vi "init.vi"(0 "Camera in":refnum<class "Camera.lvclass">, 1 "interface":u16(ring)=65535 items=["FireWire"=1, "GenICam"=3, "GigE"=5, "USB"=6, "CameraLinkME4"=7, "USB3"=8, "CLHS"=11, "All"=65535], 2 "serial":u32=4294967295 format="%0d", 3 "error in (no error)":errorcluster) -> (7 "Camera out":refnum<class "Camera.lvclass">, 10 "error out":errorcluster)   [LabVIEW 2019, in "Camera.lvclass"]
doc: "Opens communication and initializes a camera. With the \"All interfaces\" option, this VI will scan through all possible interfaces until it finds a connected camera. Alternatively, the interface can be specified. An error is generated if no camera is found. The camera is set to a defult configuration by this VI."
uses:
  Camera.lvclass
  Camera.lvclass/Camera.ctl
  pco.sdk/Structures/Structures.lvlib
  pco.sdk/CameraAccess/CameraAccess.lvlib
  pco.sdk/CameraDescription/CameraDescription.lvlib
  pco.sdk/GeneralCameraStatus/GeneralCameraStatus.lvlib
  pco.convert/Convert.lvlib
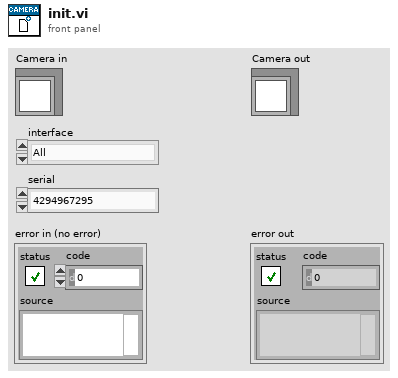
[diagram p1: front panel]
types:
  T1 = cluster{"wCamType":u16, "wCamSubType":u16, "dwSerialNumber":u32, "dwHWVersion":u32, "dwFWVersion":u32, "InterfaceType":u16, "PCO_FW_Vers":cluster{"wDeviceNum":u16, "PCO_SC2_Firmware_DESC":cluster{"szName":string, "bMinorRev":u8, "bMajorRev":u8, "wVariant":u16}[]}, "PCO_HW_Vers":cluster{"wBoardNum":u16, "PCO_SC2_Hardware_DESC":cluster{"szName":string, "wBatchNo":u16, "wRevision":u16, "wVariant":u16}[]}}
  T2 = cluster{"wSensorTypeDESC":u16, "wSensorSubTypeDESC":u16, "wMaxHorzResStdDESC":u16, "wMaxVertResStdDESC":u16, "wMaxHorzResExtDESC":u16, "wMaxVertResExtDESC":u16, "wDynResDESC":u16, "wMaxBinHorzDESC":u16, "wBinHorzSteppingDESC":u16, "wMaxBinVertDESC":u16, "wBinVertSteppingDESC":u16, "wRoiHorStepsDESC":u16, "wRoiVertStepsDESC":u16, "wNumADCsDESC":u16, "wMinSizeHorzDESC":u16, "dwPixelRateDESC":u32[], "wConvFactDESC":u16[], "sCoolingSetpoints":i16[], "wSoftRoiHorStepsDESC":u16, "wSoftRoiVertStepsDESC":u16, "wIRDESC":u16, "wMinSizeVertDESC":u16, "dwMinDelayDESC":u32, "dwMaxDelayDESC":u32, "dwMinDelayStepDESC":u32, "dwMinExposureDESC":u32, "dwMaxExposureDESC":u32, "dwMinExposureStepDESC":u32, "dwMinDelayIRDESC":u32, "dwMaxDelayIRDESC":u32, "dwMinExposureIRDESC":u32, "dwMaxExposureIRDESC":u32, "wTimeTableDESC":u16, "wDoubleImageDESC":u16, "sMinCoolSetDESC":i16, "sMaxCoolSetDESC":i16, "sDefaultCoolSetDESC":i16, "wPowerDownModeDESC":u16, "wOffsetRegulationDESC":u16, "wColorPatternDESC":u16, "wPatternTypeDESC":u16, "wNumCoolingSetpoints":u16, "dwGeneralCapsDESC1":u32, "dwGeneralCapsDESC2":u32, "dwExtSyncFrequency":u32[], "dwGeneralCapsDESC3":u32, "dwGeneralCapsDESC4":u32}
  T3 = cluster{"sharpen":bool, "adaptive_sharpen":bool, "flip_vertical":bool, "auto_minmax":bool, "add_conv_flags":u32, "min_limit":u16, "max_limit":u16, "gamma":dbl, "contrast":i32, "pco_debayer_algorithm":bool, "color_temperature":i32, "color_saturation":i32, "color_vibrance":i32, "color_tint":i32, "lut_file":path}
  T4 = cluster{"wInterfaceType":u16, "wCameraNumber":u16, "wCameraNumAtInterface":u16, "wOpenFlags":u16[], "dwOpenFlags":u32[], "wOpenPtr":u64[]}
  T5 = cluster{"iConversionFactor":i32, "iDataBits":i32, "iSensorInfoBits":i32, "iDarkOffset":i32, "strColorCoeff":dbl[], "iCamNum":i32, "hCamera":u64}
  T6 = enum16{"Undefined", "Mono8", "Mono16", "BGRA8", "RGBA8", "BGRA16", "RGBA16", "CompressedMono8"}
  T7 = map{enum16{"Undefined", "Mono8", "Mono16", "BGRA8", "RGBA8", "BGRA16", "RGBA16", "CompressedMono8"}, bool}
  T8 = map{enum16{"Undefined", "Mono8", "Mono16", "BGRA8", "RGBA8", "BGRA16", "RGBA16", "CompressedMono8"}, cluster{"sharpen":bool, "adaptive_sharpen":bool, "flip_vertical":bool, "auto_minmax":bool, "add_conv_flags":u32, "min_limit":u16, "max_limit":u16, "gamma":dbl, "contrast":i32, "pco_debayer_algorithm":bool, "color_temperature":i32, "color_saturation":i32, "color_vibrance":i32, "color_tint":i32, "lut_file":path}}
  T9 = map{enum16{"Undefined", "Mono8", "Mono16", "BGRA8", "RGBA8", "BGRA16", "RGBA16", "CompressedMono8"}, u64}
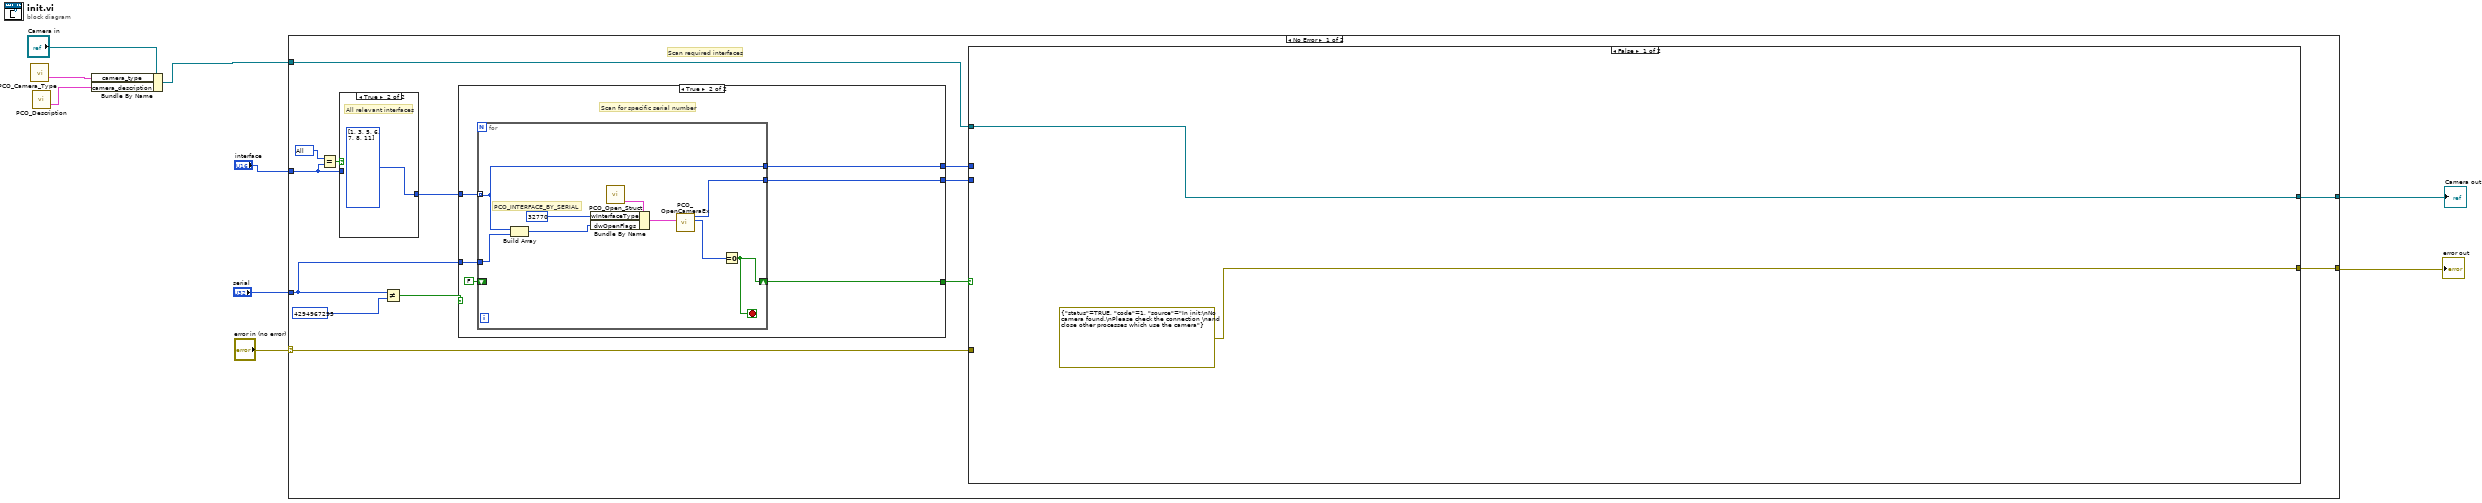
[diagram p0: block diagram]
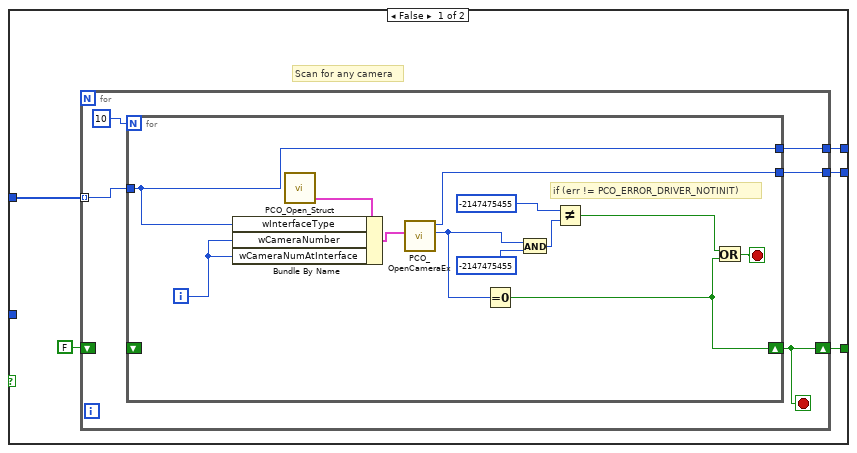
[diagram p2: hidden frame]
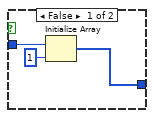
[diagram p3: hidden frame]
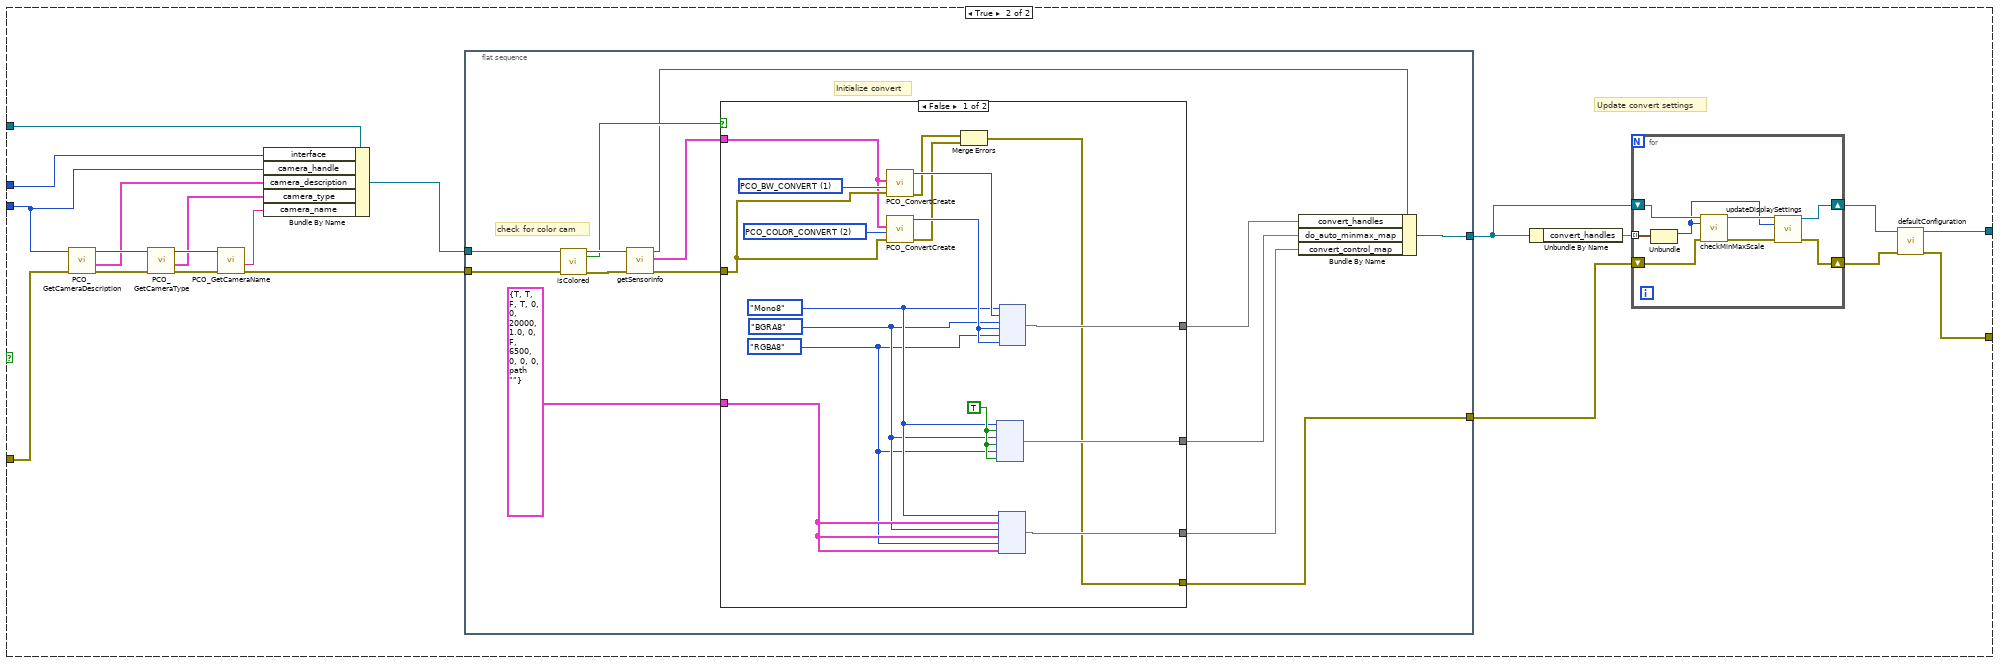
[diagram p4: hidden frame]
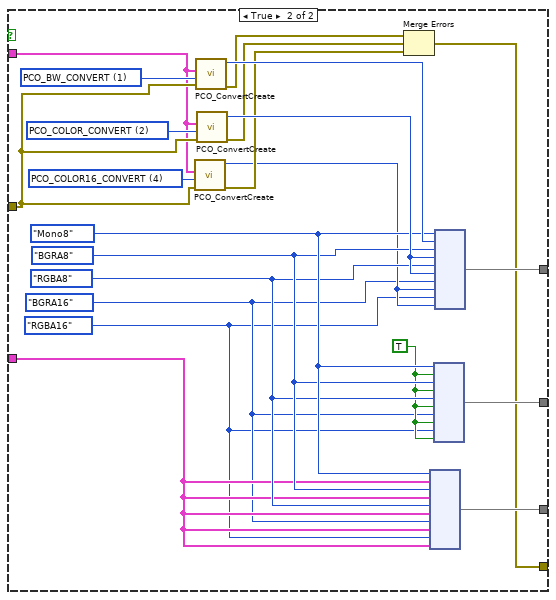
[diagram p5: hidden frame]
diagram:
  n1 = call "PCO_Camera_Type.vi"() -> ("PCO_CameraType"=w5:T1)  [unwired: 4 in, 3 out]
  n2 = call "PCO_Description.vi"() -> ("PCO_Description"=w4:T2)  [unwired: 4 in, 3 out]
  n3 = Bundle By Name(cluster="Camera in", "camera_type"=w5, "camera_description"=w4) -> (w2:refnum<class "Camera.lvclass">)
  n4 = case shown="No Error" "error in (no error)" {
    selector: "error in (no error)" -> [w15 w149]
    tunnel: [w21 w149] -> w8
    tunnel: [w19 w148] -> w7
    tunnel: w2 -> [w20 w148]
    tunnel: "interface" -> [w17 _]
    tunnel: "serial" -> [w10 _]
    frame No Error {
      w13 = u16 65535 items=["FireWire"=1, "GenICam"=3, "GigE"=5, "USB"=6, "CameraLinkME4"=7, "USB3"=8, "CLHS"=11, "All"=65535] ("interface")
      # "Scan required interfaces"
      n5 = Equal?(x=w13, y=w17) -> (x = y?=w18:bool)
      n6 = case shown="True" w18 {
        tunnel: w17 -> [w63 _]
        tunnel: [w61 u16[] [1, 3, 5, 6, 7, 8, 11]] -> w16
        frame False {
          n7 = Initialize Array(w63, 1 ("dimension size")) -> (w61:u16[])
        }
        frame True {
          # "All relevant interfaces"
        }
      }
      n8 = Not Equal?(x=w10, y=u32 4294967295) -> (x != y?=w11:bool)
      n9 = case shown="True" w11 {
        tunnel: [w28 w46] -> w23
        tunnel: [w27 w48] -> w22
        tunnel: w16 -> [w25 w50]
        tunnel: [w24 w47] -> w14
        tunnel: w10 -> [_ w49]
        frame False {
          # "Scan for any camera"
          n10 = for {
            shift-right: [w31] -> w28
            shift-left: FALSE -> [_]
            tunnel: w25 -> [w30] mode=indexing
            tunnel: [w32] -> w27
            tunnel: [w29] -> w24
            stop <- w31 stop-if-true
            n11 = for {
              N: 10 -> [_]
              tunnel: w30 -> [w34]
              shift-right: [w41] -> w31
              shift-left: _ -> [_]
              tunnel: [w39] -> w32
              tunnel: [w34] -> w29
              i -> [w35]
              stop <- w40 stop-if-true
              # "if (err != PCO_ERROR_DRIVER_NOTINIT)"
              n12 = call "PCO_Open_Struct.vi"() -> ("PCO_Open_Struct"=w45:T4)  [unwired: 4 in, 4 out]
              n13 = Bundle By Name(cluster=w45, "wInterfaceType"=w34, "wCameraNumber"=w35, "wCameraNumAtInterface"=w35) -> (w44:T4)
              n14 = call "PCO_OpenCameraEx.vi"("strOpenStruct"=w44) -> ("ErrorMessage"=w36:i32, "ph out"=w39:u64)  [unwired: 8 in, 1 out]
              n15 = Equal To 0?(x=w36) -> (x = 0?=w41:bool)
              n16 = And(x=w36, y=-2147475455 ("x")) -> (x .and. y?=w38:i32)
              n17 = Not Equal?(x=-2147475455, y=w38) -> (x != y?=w42:bool)
              n18 = Or(x=w42, y=w41) -> (x .or. y?=w40:bool)
            }
          }
        }
        frame True {
          # "Scan for specific serial number"
          n19 = for {
            shift-right: [w52] -> w46
            shift-left: FALSE -> [_]
            tunnel: w50 -> [w53] mode=indexing
            tunnel: w49 -> [w56]
            tunnel: [w54] -> w48
            tunnel: [w53] -> w47
            stop <- w52 stop-if-true
            # "PCO_INTERFACE_BY_SERIAL"
            n20 = Build Array(w53, w56) -> (w55:u32[])
            n21 = call "PCO_Open_Struct.vi"() -> ("PCO_Open_Struct"=w60:T4)  [unwired: 4 in, 4 out]
            n22 = Bundle By Name(cluster=w60, "wInterfaceType"=u16 32770, "dwOpenFlags"=w55) -> (w59:T4)
            n23 = call "PCO_OpenCameraEx.vi"("strOpenStruct"=w59) -> ("ErrorMessage"=w58:i32, "ph out"=w54:u64)  [unwired: 8 in, 1 out]
            n24 = Equal To 0?(x=w58) -> (x = 0?=w52:bool)
          }
        }
      }
      n25 = case shown="False" w23 {
        tunnel: [errorcluster {"status"=TRUE, "code"=1, "source"="In init:\nNo camera found.\nPlease check the connection \nand close other processes which use the camera"} ("error out") w69] -> w21
        tunnel: w22 -> [_ w79]
        tunnel: w20 -> [w65 w85]
        tunnel: [w65 w68] -> w19
        tunnel: w15 -> [_ w86]
        tunnel: w14 -> [_ w67]
        frame False {
        }
        frame True {
          # "Update convert settings"
          n26 = call "PCO_GetCameraDescription.vi"("error in (no error)"=w86, "ph"=w79) -> ("error out"=w84:errorcluster, "strDescription"=w80:T2, "ph out"=w83:u64)  [unwired: 6 in, 1 out]
          n27 = call "PCO_GetCameraType.vi"("error in (no error)"=w84, "ph"=w83) -> ("error out"=w81:errorcluster, "strCamType"=w78:T1, "ph out"=w82:u64)  [unwired: 6 in, 1 out]
          n28 = call "PCO_GetCameraName.vi"("error in (no error)"=w81, "ph"=w82) -> ("error out"=w76:errorcluster, "szCameraName"=w77:string)  [unwired: 6 in, 2 out]
          n29 = Bundle By Name(cluster=w85, "interface"=w67, "camera_handle"=w79, "camera_description"=w80, "camera_type"=w78, "camera_name"=w77) -> (w75:refnum<class "Camera.lvclass">)
          n30 = flat-sequence {
            tunnel: w75 -> [w108]
            tunnel: w76 -> [w107]
            tunnel: [w95] -> w73
            tunnel: [w99] -> w72
            frame #0 {
              # "check for color cam"
              # "Initialize convert"
              n31 = call-dynamic "isColored.vi"("Camera in"=w108, "error in (no error)"=w107) -> ("Camera out"=w105:refnum<class "Camera.lvclass">, "colored"=w104:bool, "error out"=w106:errorcluster)  [unwired: 11 in]
              n32 = call-dynamic "getSensorInfo.vi"("error in (no error)"=w106, "Camera in"=w105) -> ("error out"=w101:errorcluster, "PCO_SensorInfo"=w102:T5, "Camera out"=w100:refnum<class "Camera.lvclass">)  [unwired: 7 in]
              n33 = case shown="False" w104 {
                tunnel: [w124 w135] -> w98
                tunnel: [w125 w128] -> w97
                tunnel: T3 {"sharpen"=TRUE, "adaptive_sharpen"=TRUE, "flip_vertical"=FALSE, "auto_minmax"=TRUE, "add_conv_flags"=0, "min_limit"=0, "max_limit"=20000, "gamma"=1.0, "contrast"=0, "pco_debayer_algorithm"=FALSE, "color_temperature"=6500, "color_saturation"=0, "color_vibrance"=0, "color_tint"=0, "lut_file"=path ""} ("convert_control") -> [w122 w134]
                tunnel: [w123 w127] -> w96
                tunnel: w102 -> [w117 w136]
                tunnel: w101 -> [w118 w137]
                tunnel: [w109 w126] -> w95
                frame False {
                  w110 = T6."RGBA8" ("data_format")
                  w111 = T6."BGRA8" ("data_format")
                  w112 = T6."Mono8" ("data_format")
                  w121 = TRUE
                  w119 = 2 items=["PCO_BW_CONVERT"=1, "PCO_COLOR_CONVERT"=2, "PCO_PSEUDO_CONVERT"=3, "PCO_COLOR16_CONVERT"=4]
                  w120 = 1 items=["PCO_BW_CONVERT"=1, "PCO_COLOR_CONVERT"=2, "PCO_PSEUDO_CONVERT"=3, "PCO_COLOR16_CONVERT"=4]
                  n34 = call "PCO_ConvertCreate.vi"("error in (no error)"=w118, "iConvertType"=w120, "strSensor"=w117) -> ("error out"=w114:errorcluster, "ph out"=w116:u64)  [unwired: 6 in, 1 out]
                  n35 = call "PCO_ConvertCreate.vi"("error in (no error)"=w118, "iConvertType"=w119, "strSensor"=w117) -> ("error out"=w113:errorcluster, "ph out"=w115:u64)  [unwired: 6 in, 1 out]
                  n36 = Merge Errors(w114, w113) -> (w109:errorcluster)
                  n37 = node(w112, w121, w111, w121, w110, w121) -> (w125:T7)
                  n38 = node(w112, w122, w111, w122, w110, w122) -> (w123:T8)
                  n39 = node(w112, w116, w111, w115, w110, w115) -> (w124:T9)
                }
                frame True {
                  w129 = T6."RGBA16" ("data_format")
                  w130 = T6."BGRA16" ("data_format")
                  w138 = 4 items=["PCO_BW_CONVERT"=1, "PCO_COLOR_CONVERT"=2, "PCO_PSEUDO_CONVERT"=3, "PCO_COLOR16_CONVERT"=4]
                  w139 = T6."RGBA8" ("data_format")
                  w140 = T6."BGRA8" ("data_format")
                  w141 = T6."Mono8" ("data_format")
                  w133 = TRUE
                  w146 = 2 items=["PCO_BW_CONVERT"=1, "PCO_COLOR_CONVERT"=2, "PCO_PSEUDO_CONVERT"=3, "PCO_COLOR16_CONVERT"=4]
                  w147 = 1 items=["PCO_BW_CONVERT"=1, "PCO_COLOR_CONVERT"=2, "PCO_PSEUDO_CONVERT"=3, "PCO_COLOR16_CONVERT"=4]
                  n40 = call "PCO_ConvertCreate.vi"("error in (no error)"=w137, "iConvertType"=w138, "strSensor"=w136) -> ("error out"=w132:errorcluster, "ph out"=w131:u64)  [unwired: 6 in, 1 out]
                  n41 = call "PCO_ConvertCreate.vi"("error in (no error)"=w137, "iConvertType"=w147, "strSensor"=w136) -> ("error out"=w143:errorcluster, "ph out"=w145:u64)  [unwired: 6 in, 1 out]
                  n42 = call "PCO_ConvertCreate.vi"("error in (no error)"=w137, "iConvertType"=w146, "strSensor"=w136) -> ("error out"=w142:errorcluster, "ph out"=w144:u64)  [unwired: 6 in, 1 out]
                  n43 = Merge Errors(w143, w142, w132) -> (w126:errorcluster)
                  n44 = node(w141, w134, w140, w134, w139, w134, w130, w134, w129, w134) -> (w127:T8)
                  n45 = node(w141, w133, w140, w133, w139, w133, w130, w133, w129, w133) -> (w128:T7)
                  n46 = node(w141, w145, w140, w144, w139, w144, w130, w131, w129, w131) -> (w135:T9)
                }
              }
              n47 = Bundle By Name(cluster=w100, "convert_handles"=w98, "do_auto_minmax_map"=w97, "convert_control_map"=w96) -> (w99:refnum<class "Camera.lvclass">)
            }
          }
          n48 = Unbundle By Name(w72) -> ("convert_handles"=w74:T9)
          n49 = for {
            tunnel: w74 -> [w94] mode=indexing
            shift-right: [w93] -> w71
            shift-left: w72 -> [w91]
            shift-right: [w92] -> w70
            shift-left: w73 -> [w89]
            n50 = Unbundle(w94) -> (w87:T6)  [unwired: 1 out]
            n51 = call-dynamic "checkMinMaxScale.vi"("Camera in"=w91, "data_format"=w87, "error in (no error)"=w89) -> ("Camera out"=w90:refnum<class "Camera.lvclass">, "error out"=w88:errorcluster)  [unwired: 10 in, 1 out]
            n52 = call-dynamic "updateDisplaySettings.vi"("Camera in"=w90, "data_format"=w87, "error in (no error)"=w88) -> ("Camera out"=w93:refnum<class "Camera.lvclass">, "error out"=w92:errorcluster)  [unwired: 11 in]
          }
          n53 = call-dynamic "defaultConfiguration.vi"("error in (no error)"=w70, "Camera in"=w71) -> ("error out"=w69:errorcluster, "Camera out"=w68:refnum<class "Camera.lvclass">)  [unwired: 8 in]
        }
      }
    }
    frame Error {
    }
  }
  "error out" <- w8
  "Camera out" <- w7
